vi "4.7.vi"() -> ()   [LabVIEW 2017]
panel:
  out "循环次数":dbl
  out "随机数":dbl
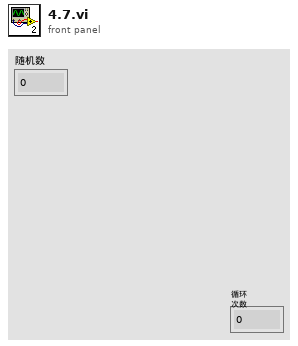
[diagram p1: front panel]
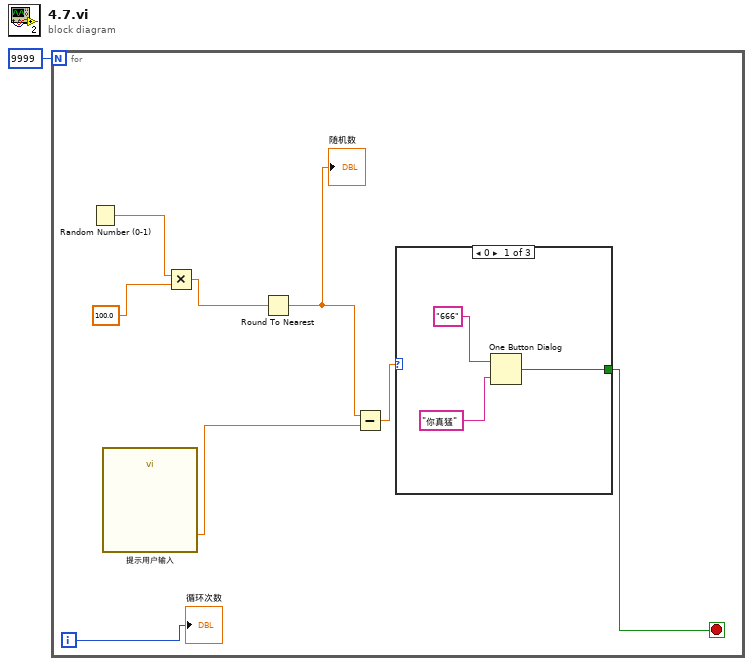
[diagram p0: block diagram]
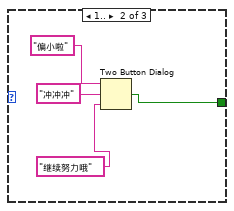
[diagram p2: hidden frame]
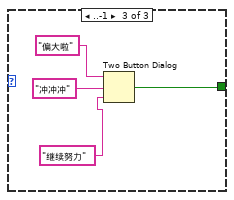
[diagram p3: hidden frame]
diagram:
  n1 = for {
    N: 9999 -> [_]
    i -> [w6]
    stop <- w5 stop-if-true
    n2 = Random Number (0-1)() -> (number: 0 to 1=w9:dbl)
    n3 = call "提示用户输入"() -> ("请在1-1000猜"=w4:dbl)  [unwired: 17 in, 2 out]
    n4 = Multiply(x=w9, y=100.0) -> (x*y=w3:dbl)
    n5 = Round To Nearest(number=w3) -> (nearest integer value=w2:dbl)
    "随机数" <- w2
    n6 = Subtract(x=w2, y=w4) -> (x-y=w7:dbl)
    n7 = case shown="0" w7 {
      tunnel: [w12 w13 w17] -> w5
      frame 0 {
        n8 = One Button Dialog(message="666", button name ("OK")="你真猛") -> (true=w12:bool)
      }
      frame 1.. {
        n9 = Two Button Dialog(message="偏小啦", 1:"继续努力哦", 2:"冲冲冲") -> (T button?=w13:bool)
      }
      frame ..-1 {
        n10 = Two Button Dialog(message="偏大啦", 1:"继续努力", 2:"冲冲冲") -> (T button?=w17:bool)
      }
    }
    "循环次数" <- w6
  }
